vi "CLD 6 CSV file utility.vi"(8 "Error In":errorcluster, 9 "Path":path, 10 "[Data In]":T1[](array[typedef])=[{"Dwell Time"=3, "State 1"=TRUE, "State 2"=FALSE, "State 3"=FALSE}, {"Dwell Time"=4, "State 1"=FALSE, "State 2"=TRUE, "State 3"=FALSE}, {"Dwell Time"=5, "State 1"=FALSE, "State 2"=FALSE, "State 3"=TRUE}], 11 "CLD 6 file Enum":T2) -> (0 "Error Out":errorcluster, 3 "[Data Out]":T1[](array[typedef]))   [LabVIEW 2018]
doc: "CLD 6 exercise"
uses:
  CLD 6 CSV file enum.ctl
  CLD 6 CSV file data structure.ctl
  <vilib>/Utility/file.llb/Read Delimited Spreadsheet (string).vi
  <vilib>/Utility/file.llb/Write Delimited Spreadsheet (string).vi
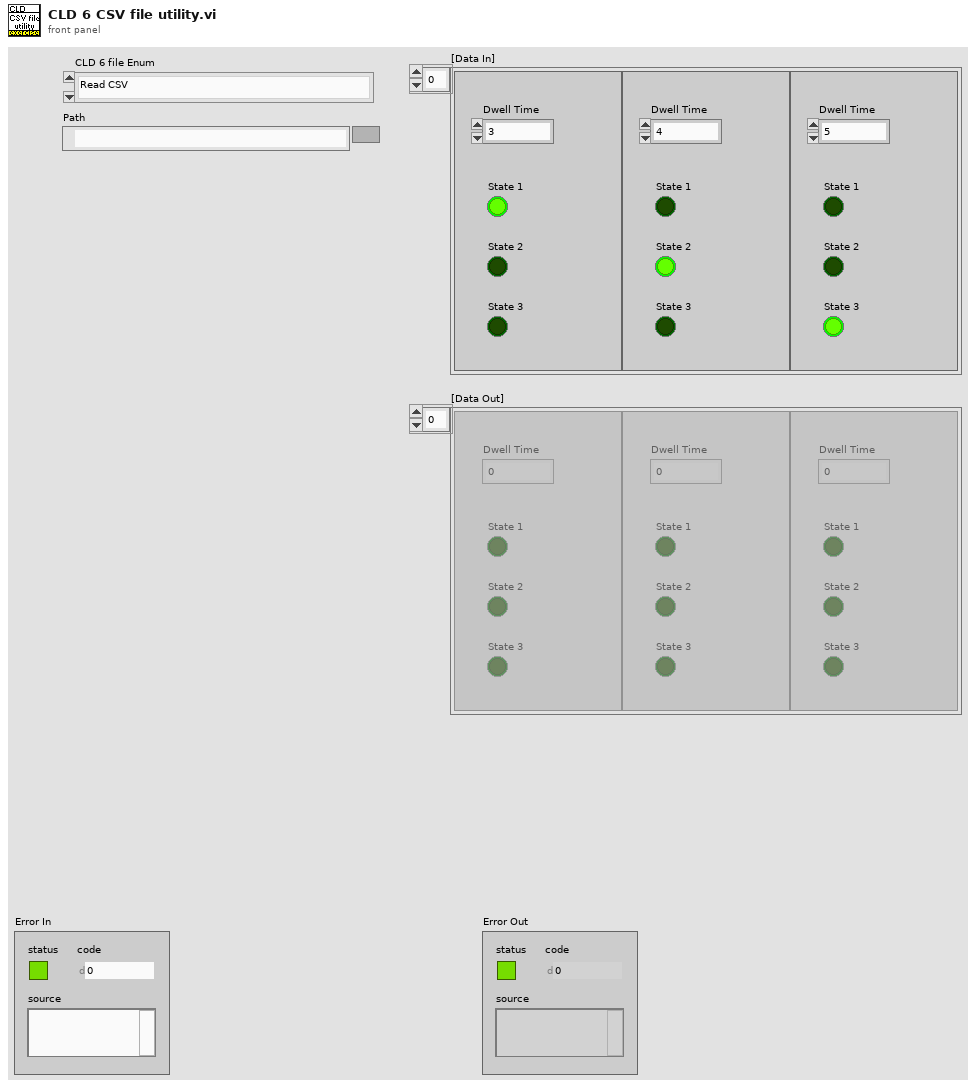
[diagram p1: front panel]
types:
  T1 = typedef "CLD 6 CSV file data structure.ctl" = cluster{"Dwell Time":i32, "State 1":bool, "State 2":bool, "State 3":bool}
  T2 = typedef "CLD 6 CSV file enum.ctl" = enum16{"Read CSV", "Write CSV"}
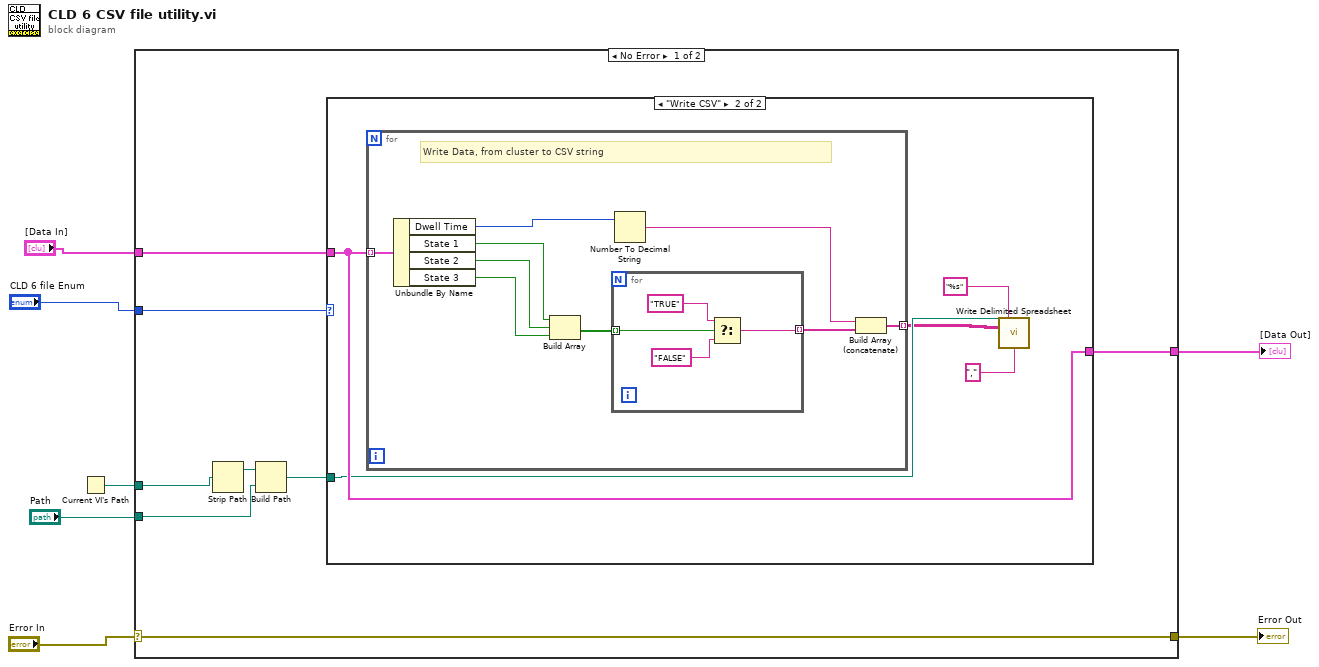
[diagram p0: block diagram]
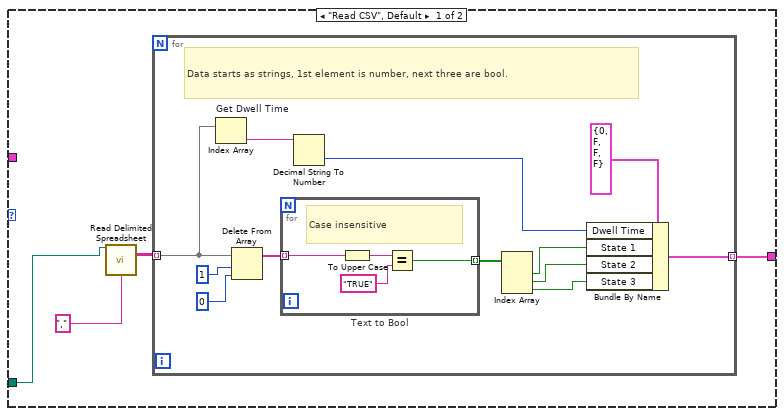
[diagram p2: hidden frame]
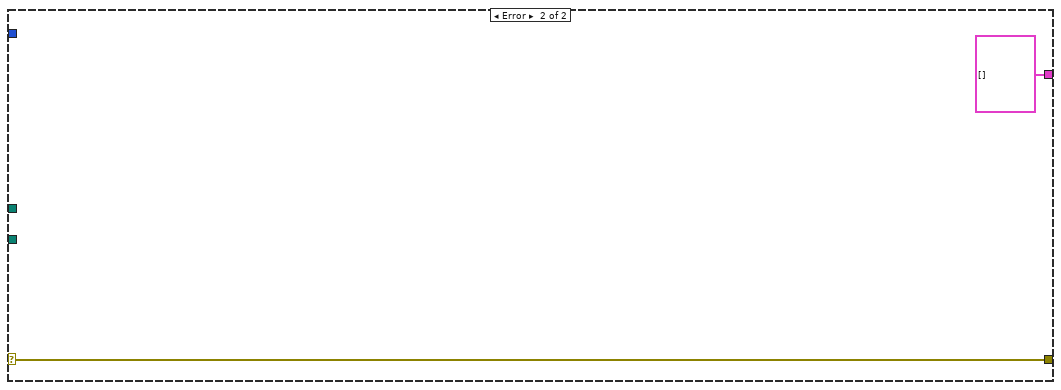
[diagram p3: hidden frame]
diagram:
  n1 = Current VI's Path() -> (path=w7:path)
  n2 = case shown="No Error" "Error In" {
    selector: "Error In" -> [w9 w55]
    tunnel: [w15 T1[] [] ("[Data In]")] -> w4
    tunnel: "Path" -> [w14 _]
    tunnel: w7 -> [w13 _]
    tunnel: "CLD 6 file Enum" -> [w11 _]
    tunnel: "[Data In]" -> [w10 _]
    tunnel: [w9 w55] -> w1
    frame No Error {
      n3 = Strip Path(path=w13) -> (stripped path=w8:path)  [unwired: 1 out]
      n4 = Build Path(base path=w8, name or relative path=w14) -> (appended path=w12:path)
      n5 = case shown="\"Write CSV\"" w11 {
        tunnel: w12 -> [w17 w38]
        tunnel: [w19 w40] -> w15
        tunnel: w10 -> [_ w40]
        frame "Read CSV", Default {
          n6 = call-poly <vilib>:"Read Delimited Spreadsheet.vi"("file path (dialog if empty)"=w17, "delimiter (\\t)"="," ("delimiter (\\t)")) -> ("all rows"=w18:string[][])  [unwired: 8 in, 5 out]
          n7 = for {
            tunnel: w18 -> [w28] mode=indexing
            tunnel: [w31] -> w19 mode=indexing
            # "Data starts as strings, 1st element is number, next three are bool."
            n8 = Index Array "Get Dwell Time"(array=w28) -> (element=w30:string)  [unwired: 1 in]
            n9 = Delete From Array(array=w28, length=1, index=0) -> (array with subset deleted=w21:string[])  [unwired: 1 out]
            n10 = for "Text to Bool" {
              tunnel: w21 -> [w35] mode=indexing
              tunnel: [w32] -> w25 mode=indexing
              # "Case insensitive"
              n11 = To Upper Case(1:w35) -> (0:w34:string)
              n12 = Equal?(x=w34, y="TRUE") -> (x = y?=w32:bool)
            }
            n13 = Decimal String To Number(string=w30) -> (number=w29:i32)  [unwired: 2 in, 1 out]
            n14 = Index Array(array=w25) -> (element #1=w24:bool, element #2=w23:bool, element #3=w22:bool)  [unwired: 3 in]
            n15 = Bundle By Name(cluster=T1 {"Dwell Time"=0, "State 1"=FALSE, "State 2"=FALSE, "State 3"=FALSE} ("CSV File Data Structure"), "Dwell Time"=w29, "State 1"=w24, "State 2"=w23, "State 3"=w22) -> (w31:T1)
          }
        }
        frame "Write CSV" {
          n16 = for {
            tunnel: w40 -> [w49] mode=indexing
            tunnel: [w41] -> w37 mode=indexing
            # "Write Data, from cluster to CSV string"
            n17 = Unbundle By Name(w49) -> ("Dwell Time"=w48:i32, "State 1"=w47:bool, "State 2"=w46:bool, "State 3"=w45:bool)
            n18 = Build Array(w47, w46, w45) -> (w44:bool[])
            n19 = for {
              tunnel: w44 -> [w53] mode=indexing
              tunnel: [w50] -> w42 mode=indexing
              n20 = Select(t="TRUE", s=w53, f="FALSE") -> (s? t:f=w50:string)
            }
            n21 = Number To Decimal String(number=w48) -> (decimal integer string=w43:string)  [unwired: 1 in]
            n22 = Build Array (concatenate)(w43, w42) -> (w41:string[])
          }
          n23 = call-poly <vilib>:"Write Delimited Spreadsheet.vi"("file path (dialog if empty)"=w38, "format (%s)"="%s", "2D data"=w37, "delimiter (\\t)"="," ("delimiter (\\t)")) -> ()  [unwired: 10 in, 2 out]
        }
      }
    }
    frame Error {
    }
  }
  "[Data Out]" <- w4
  "Error Out" <- w1
